vi "GetBgColorFromBoolCtrl.vi"(11 "bool ref in":refnum<vi>) -> (2 "bg color":u32(colorbox)=65280, 3 "bool ref out":refnum<vi>)   [LabVIEW 2018, in "Library-Ctrl.lvlib"]
uses:
  Library-Ctrl.lvlib
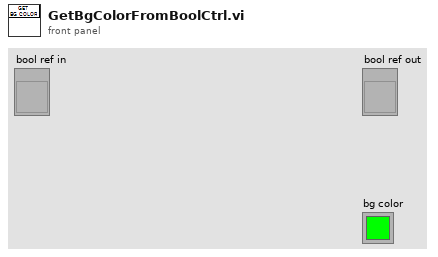
[diagram p1: front panel]
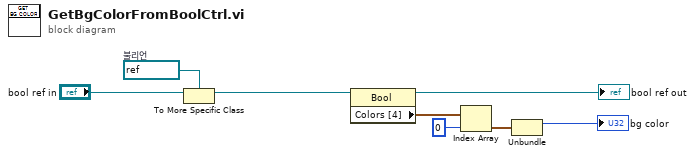
[diagram p0: block diagram]
diagram:
  w6 = refnum<vi> refnum  # 불리언
  n1 = To More Specific Class(target class=w6, reference="bool ref in") -> (specific class reference=w7:refnum<vi>)  [unwired: 1 in, 1 out]
  n2 = property class="Bool"(reference=w7) -> (reference out=→"bool ref out":refnum<vi>, "Colors [4]"=w5:cluster{u32, u32}[])  [unwired: 1 in, 1 out]
  n3 = Index Array(array=w5, index=0 ("인덱스")) -> (element=w3:cluster{u32, u32})
  n4 = Unbundle(w3) -> (→"bg color":u32)  [unwired: 1 out]
